vi "Port Index Search.vi"(8 "error in":errorcluster) -> (0 "error out":errorcluster, 1 "Decimal Port Index":i32, 2 "Port Index":string, 3 "Device Description":string)   [LabVIEW 2022 SP3]
panel:
  out "Array":string[](array[string])
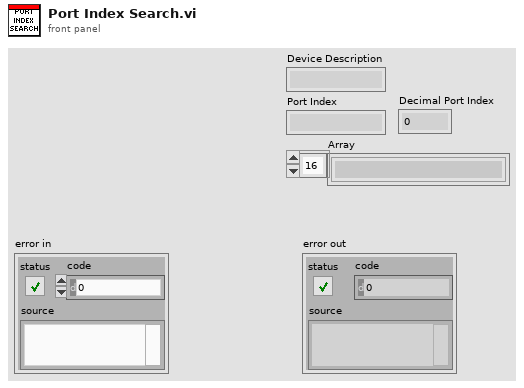
[diagram p1: front panel]
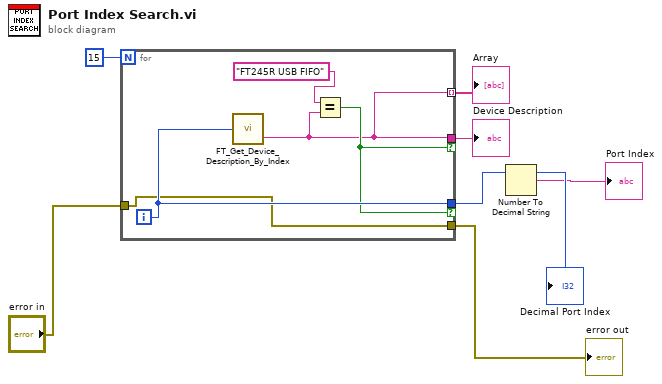
[diagram p0: block diagram]
diagram:
  n1 = for {
    N: 15 -> [_]
    tunnel: [w8] -> w6 if=w10
    tunnel: [w11] -> w5 if=w10
    tunnel: "error in" -> [w9]
    tunnel: [w9] -> w1
    tunnel: [w8] -> w2 mode=indexing
    i -> [w11]
    n2 = call "FT_Get_Device_Description_By_Index.vi"("Device Index"=w11) -> ("Device Description"=w8:string)  [unwired: 1 out]
    n3 = Equal?(x="FT245R USB FIFO", y=w8) -> (x = y?=w10:bool)
  }
  "Device Description" <- w6
  "error out" <- w1
  "Array" <- w2
  "Decimal Port Index" <- w5
  n4 = Number To Decimal String(number=w5) -> (decimal integer string=→"Port Index":string)  [unwired: 1 in]
